vi "ClientSDO_readU8.vi"(8 "error in (no error)":errorcluster, 9 "sub_index":u8, 10 "object_index":u16, 11 "ClientSDO Ref in":refnum<k24>) -> (0 "error IO":errorcluster, 1 "ErrorCode":u32, 2 "val":u8, 3 "ClientSDO Ref out":refnum<k24>, 4 "objectRead":i32)   [LabVIEW 2011, in "CANOpen.lvlib"]
doc: "read a byte from client using SDO protocol"
uses:
  CANOpen.lvlib
  D:/Inteliss/imt_test_app/canopenlib_cli.dll
  canopenlib_cli.dll
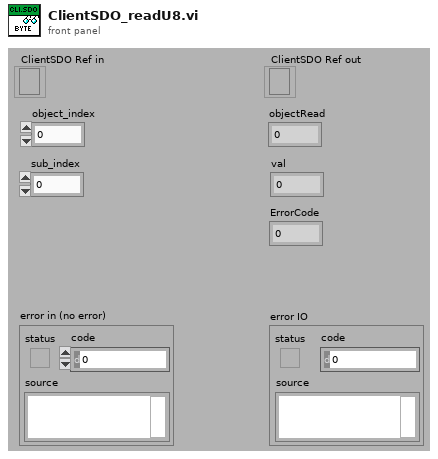
[diagram p1: front panel]
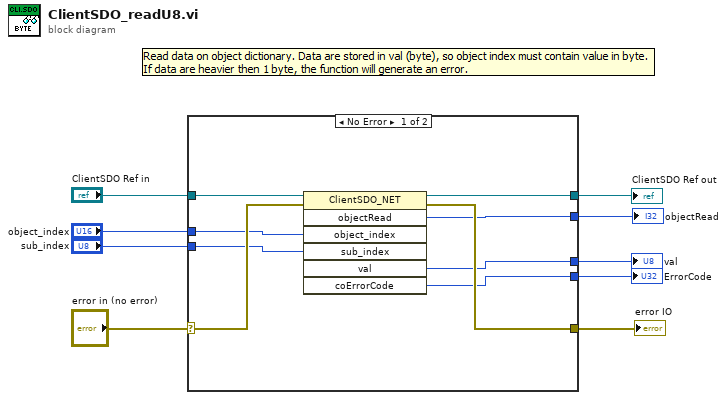
[diagram p0: block diagram]
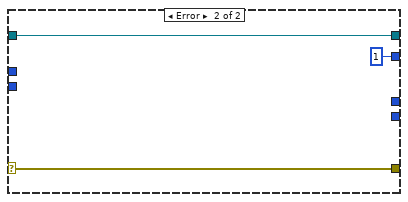
[diagram p2: hidden frame]
diagram:
  n1 = case shown="No Error" "error in (no error)" {
    selector: "error in (no error)" -> [w17 w20]
    tunnel: "ClientSDO Ref in" -> [w18 w21]
    tunnel: "object_index" -> [w16 _]
    tunnel: "sub_index" -> [w15 _]
    tunnel: [w14 w21] -> w5
    tunnel: [w13 w20] -> w2
    tunnel: [w12 _] -> w4
    tunnel: [w11 _] -> w3
    tunnel: [w10 1 ("objectRead")] -> w1
    frame No Error {
      n2 = invoke class="ClientSDO_NET" method="objectRead"(reference=w18, error in=w17, "object_index"=w16, "sub_index"=w15) -> (reference out=w14:refnum<k24>, error out=w13:errorcluster, "objectRead"=w10:i32, "val"=w12:u8, "coErrorCode"=w11:u32)  [unwired: 3 in, 2 out]
    }
    frame Error {
    }
  }
  "ClientSDO Ref out" <- w5
  "val" <- w4
  "ErrorCode" <- w3
  "error IO" <- w2
  "objectRead" <- w1
